vi "Get Tables.vi"(8 "error in (no error)":errorcluster, 10 "System Tables (F)":bool, 11 "ODBC in":refnum<class "ADODB.lvclass">) -> (0 "error out":errorcluster, 2 "Table Names":string[](array[string]), 3 "ODBC out":refnum<class "ADODB.lvclass">)   [LabVIEW 2020, in "ADODB.lvclass"]
uses:
  ADODB.lvclass
  ADODB.lvclass/ADODB.ctl
  <vilib>/addons/database/NI_Database_API.lvlib
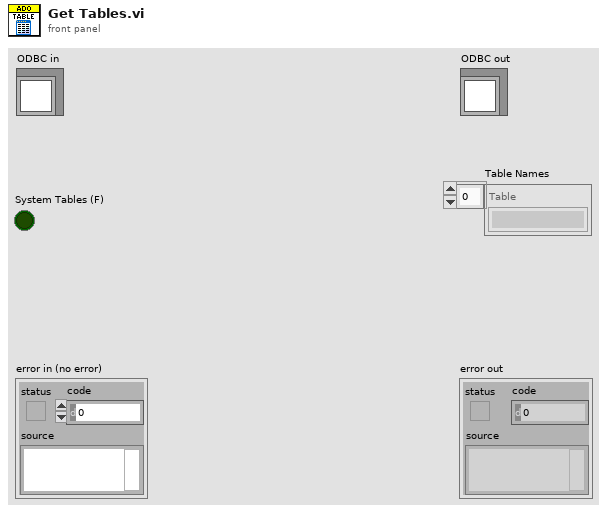
[diagram p1: front panel]
types:
  T1 = typedef "NI_Database_API.lvlib/Conn ObjectReference.ctl" = refnum<k1>
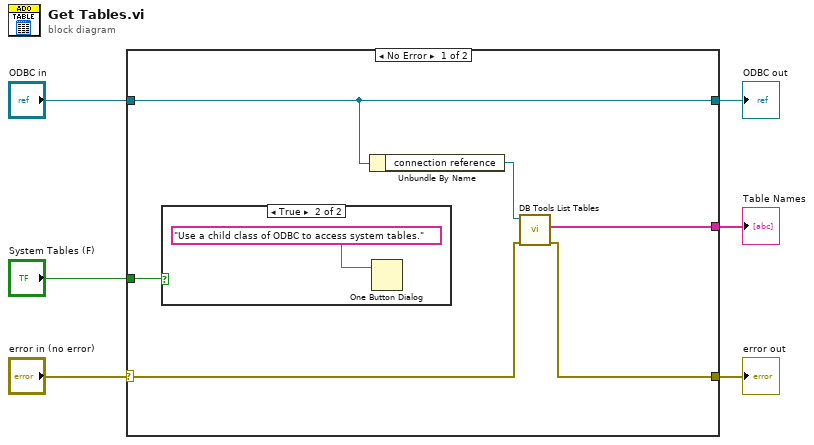
[diagram p0: block diagram]
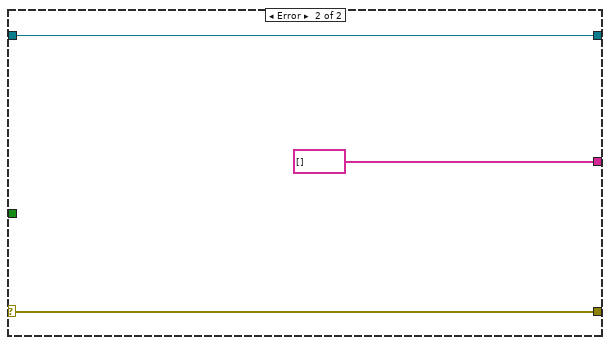
[diagram p3: hidden frame]
diagram:
  n1 = case shown="No Error" "error in (no error)" {
    selector: "error in (no error)" -> [w9 w16]
    tunnel: [w8 w16] -> w5
    tunnel: "ODBC in" -> [w11 w15]
    tunnel: [w11 w15] -> w3
    tunnel: [w12 string[] [] ("Table Names")] -> w2
    tunnel: "System Tables (F)" -> [w7 _]
    frame No Error {
      n2 = case shown="True" w7 {
        frame False {
        }
        frame True {
          n3 = One Button Dialog(message="Use a child class of ODBC to access system tables.") -> ()  [unwired: 1 in, 1 out]
        }
      }
      n4 = Unbundle By Name(w11) -> ("connection reference"=w10:T1)
      n5 = call <vilib>:"DB Tools List Tables.vi"("error in (no error)"=w9, "connection reference"=w10) -> ("error out"=w8:errorcluster, "tables"=w12:string[])  [unwired: 3 in, 1 out]
    }
    frame Error {
    }
  }
  "error out" <- w5
  "ODBC out" <- w3
  "Table Names" <- w2
